vi "Append to Binary File.vi"(0 "file path":path, 7 "data":dbl[](array[numeric]), 11 "error in (no error)":errorcluster) -> (4 "file path out":path, 15 "error out":errorcluster)   [LabVIEW 2020]
doc: "Appends text to the end of a file. Creates the file if it doesn't exist."
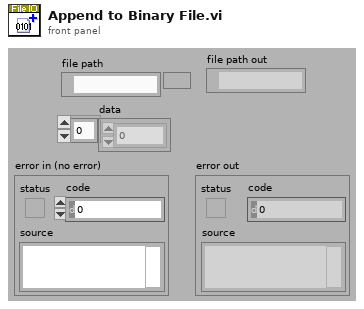
[diagram p1: front panel]
types:
  T1 = enum16{"big-endian, network order", "native, host order", "little-endian"}
  T2 = enum16{"open", "replace", "create", "open or create", "replace or create", "replace or create with confirmation"}
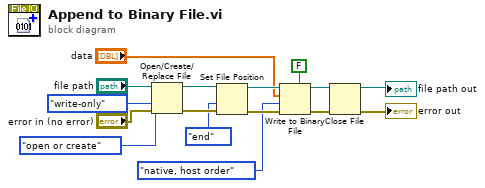
[diagram p0: block diagram]
diagram:
  n1 = Open/Create/Replace File(file path (use dialog)="file path", error in="error in (no error)", operation (0:open)=T2."open or create", access (0:read/write)=enum16{"read/write", "read-only", "write-only"}."write-only") -> (refnum out=w12:refnum<file>, error out=w13:errorcluster)  [unwired: 2 in, 1 out]
  n2 = Set File Position(refnum=w12, from (0:start)=enum16{"start", "end", "current"}."end", error in=w13) -> (refnum out=w10:refnum<file>, error out=w11:errorcluster)  [unwired: 1 in]
  n3 = Write to Binary File(file (use dialog)=w10, data="data", error in=w11, 5:FALSE ("prepend array or string size? (T)"), 9:T1."native, host order" ("byte order (0:big-endian, network order)")) -> (refnum out=w7:refnum<file>, error out=w8:errorcluster)  [unwired: 1 in, 1 out]
  n4 = Close File(refnum=w7, error in=w8) -> (path=→"file path out":path, error out=→"error out":errorcluster)
